vi "Refresh Channel Data.vi"(8 "error in (no error)":errorcluster, 11 "CIFChannelMng in":refnum<class "CIFChannelMng.lvclass">) -> (0 "error out":errorcluster, 3 "CIFChannelMng out":refnum<class "CIFChannelMng.lvclass">)   [LabVIEW 2021, in "CIFChannelMng.lvclass"]
uses:
  CIFChannelMng.lvclass
  CIFChannelMng.lvclass/CIFChannelMng.ctl
  <vilib>/CIF Foundation/CIF CIPC/TypeDefs/Read Configuration.ctl
  <vilib>/CIF Foundation/CIF CIPC/TypeDefs/Read Position.ctl
  typedef/TX CIPC Data.ctl
  typedef/TX Commands.ctl
  8bba354e-317d-4116-a685-ab5cd7060b87.vi
  <vilib>/CIF Foundation/CIF CIPC/SubVIs/Wait For N Elements Available.vi
  <vilib>/CIF Foundation/CIF CIPC/SubVIs/Check Error.vi
  <vilib>/CIF Foundation/CIF CIPC/SubVIs/Get dll Path.vi
  <vilib>/CIF Foundation/CIF CIPC/SubVIs/Get Element Read Position.vi
  <vilib>/CIF Foundation/CIF CIPC/SubVIs/Set Element Read Position.vi
  <vilib>/CIF Foundation/CIF CIPC/SubVIs/Get Element Info Variant.vi
  <vilib>/CIF Foundation/CIF CIPC/SubVIs/Check Error Core.vi
  <vilib>/CIF Foundation/CIF CIPC/CIF_NI_CIPC.lvlib
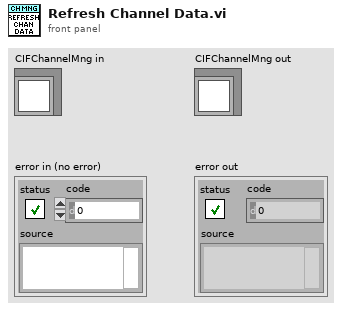
[diagram p1: front panel]
types:
  T1 = typedef "CIF_NI_CIPC.lvlib/Read Configuration.ctl" = cluster{"Read Position":T2, "Element Offset":i32, "Prepend Array Size":bool, "Get Read Position":bool}
  T2 = typedef "CIF_NI_CIPC.lvlib/Read Position.ctl" = enum8{"Next", "Newest", "Oldest", "Next Available", "Absolute"}
  T3 = typedef "CIFChannelMng.lvclass/TX CIPC Data.ctl" = cluster{"TX Commands":T4}
  T4 = typedef "CIFChannelMng.lvclass/TX Commands.ctl" = enum8{"Channel List", "New FIFO Pub"}
  T5 = typedef "CIFChannelMng.lvclass/Channel List for OOB.ctl" = cluster{"Name":string, "Direction":T6, "Type":string, "Connected?":bool, "Connected Name":string, "Custom Config Data":u8[], "Forced?":bool, "Pattern":T7}
  T6 = typedef "CIFChannels.lvclass/Direction.ctl" = enum8{"Publisher", "Subscriber"}
  T7 = typedef "ChannelCommon.lvlib/Channel Pattern.ctl" = enum8{"Unknown", "Tag", "FIFO", "MultiFIFO", "BackpressureFIFO"}
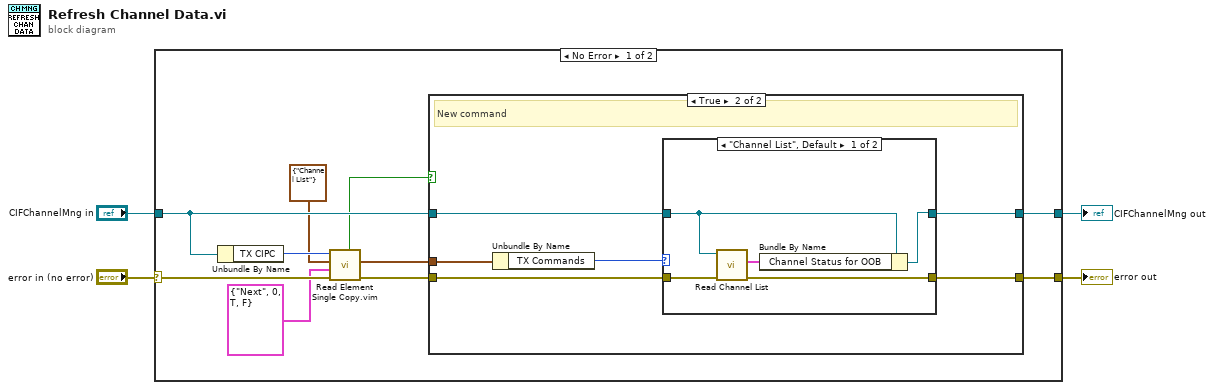
[diagram p0: block diagram]
diagram:
  n1 = case shown="No Error" "error in (no error)" {
    selector: "error in (no error)" -> [w11 w30]
    tunnel: "CIFChannelMng in" -> [w13 w31]
    tunnel: [w14 w30] -> w1
    tunnel: [w5 w31] -> w2
    frame No Error {
      n2 = Unbundle By Name(w13) -> ("TX CIPC"=w12:u64)
      n3 = call "Read Element Single Copy.vim"("error in (no error)"=w11, "Read Configuration"=T1 {"Read Position"=enum."Next", "Element Offset"=0, "Prepend Array Size"=TRUE, "Get Read Position"=FALSE}, "Data in"=T3 {"TX Commands"=enum."Channel List"} ("TX CIPC Data"), "CIPC Reference in"=w12) -> ("error out"=w9:errorcluster, "Data out"=w6:T3, "Success"=w8:bool)  [unwired: 3 in, 2 out]
      n4 = case shown="True" w8 {
        tunnel: w6 -> [_ w18]
        tunnel: w9 -> [w16 w22]
        tunnel: [w16 w21] -> w14
        tunnel: w13 -> [w15 w20]
        tunnel: [w15 w19] -> w5
        frame False {
          # "No return message yet."
        }
        frame True {
          # "New command"
          n5 = Unbundle By Name(w18) -> ("TX Commands"=w17:T4)
          n6 = case shown="\"Channel List\", Default" w17 {
            tunnel: w22 -> [w27 w28]
            tunnel: [w26 w28] -> w21
            tunnel: [w24 w29] -> w19
            tunnel: w20 -> [w23 w29]
            frame "Channel List", Default {
              n7 = call "Read Channel List.vi"("error in"=w27, "CIFChannelMng in"=w23) -> ("error out"=w26:errorcluster, "Channel List"=w25:T5[])  [unwired: 7 in, 1 out]
              n8 = Bundle By Name(cluster=w23, "Channel Status for OOB"=w25) -> (w24:refnum<class "CIFChannelMng.lvclass">)
            }
            frame "New FIFO Pub" {
              # "Could add warning"
              # "This case should not happen"
            }
          }
        }
      }
    }
    frame Error {
    }
  }
  "error out" <- w1
  "CIFChannelMng out" <- w2
